vi "6229_init_)test.vi"(0 "Atom Shutter":bool) -> ()   [LabVIEW 2015]
uses:
  <vilib>/DAQmx/write.llb/DAQmx Write.vi
  <vilib>/DAQmx/write.llb/DAQmx Write (Digital Bool 1Line 1Point).vi
  <vilib>/DAQmx/create/channels.llb/DAQmx Create Channel (DO-Digital Output).vi
  <vilib>/DAQmx/miscellaneous.llb/DAQmx Fill In Error Info.vi
panel:
  out "error out":errorcluster
  in  "Control Port":tag="6221_IR_ODT/port0/line0"
  in  "error in":errorcluster
  # "OFF"
  # "ON"
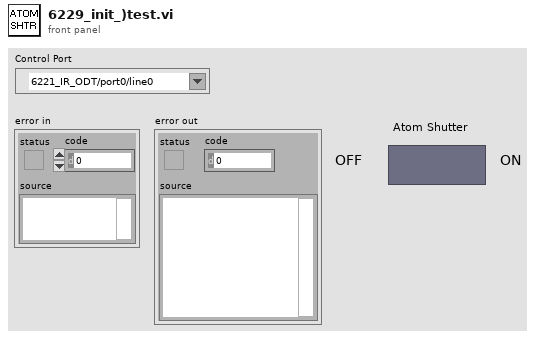
[diagram p1: front panel]
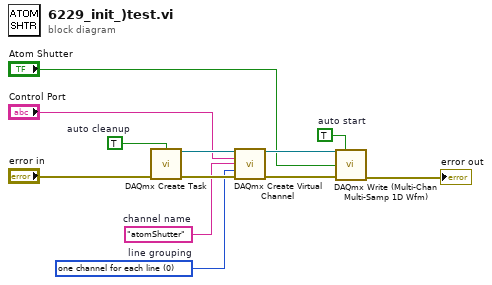
[diagram p0: block diagram]
diagram:
  w8 = 0 items=["one channel for each line", "one channel for all lines"]  # line grouping
  w7 = "atomShutter"  # channel name
  w9 = TRUE  # auto cleanup
  w12 = TRUE  # auto start
  n1 = call <vilib>:"DAQmx Create Task.vi"("auto cleanup"=w9, "error in"="error in") -> ("task out"=w6:refnum<k21>, "error out"=w10:errorcluster)  [unwired: 12 in]
  n2 = call-poly <vilib>:"DAQmx Create Virtual Channel.vi"("task in"=w6, "lines"="Control Port", "name to assign"=w7, "line grouping"=w8, "error in"=w10) -> ("task out"=w3:refnum<k21>, "error out"=w2:errorcluster)  [unwired: 9 in]
  n3 = call-poly "DAQmx Write (Multi-Chan Multi-Samp 1D Wfm).vi"("task/channels in"=w3, "auto start"=w12, "data"="Atom Shutter", "error in"=w2) -> ("error out"=→"error out":errorcluster)  [unwired: 9 in, 2 out]
